vi "ALR ON_OFFs.vi"(8 "error in (no error)":errorcluster, 9 "Data":bool[](array[boolean]), 10 "Index":i32[](array[numeric]), 11 "ALR_ON_OFF":T1) -> (0 "error out":errorcluster, 3 "ALR_ON_OFF out":T1)   [LabVIEW 2019, in "Alarms.lvlib"]
uses:
  Alarms.lvlib
  Ctl/ALR_ON_OFF.ctl
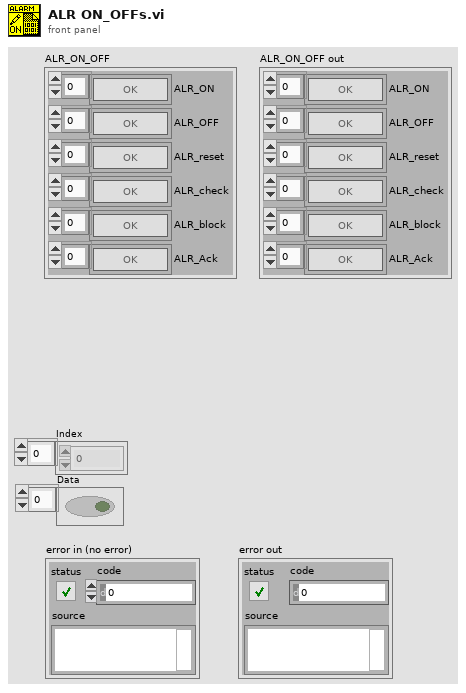
[diagram p1: front panel]
types:
  T1 = typedef "Alarms.lvlib/ALR_ON_OFF.ctl" = cluster{"ALR_ON":bool[], "ALR_OFF":bool[], "ALR_reset":bool[], "ALR_check":bool[], "ALR_block":bool[], "ALR_Ack":bool[]}
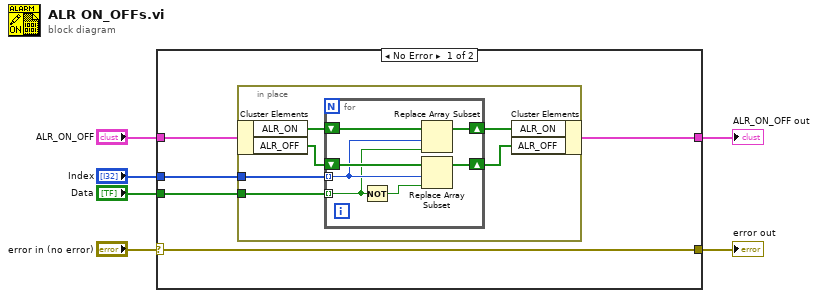
[diagram p0: block diagram]
diagram:
  n1 = case shown="No Error" "error in (no error)" {
    selector: "error in (no error)" -> [w8 w26]
    tunnel: "Index" -> [w11 _]
    tunnel: [w8 w26] -> w5
    tunnel: "ALR_ON_OFF" -> [w9 w25]
    tunnel: "Data" -> [w10 _]
    tunnel: [w7 w25] -> w1
    frame No Error {
      n2 = in-place {
        in-place-border: w11 -> [w16]
        in-place-border: w10 -> [w14]
        n3 = in-place-cluster #1(w9) -> ("ALR_ON"=w17:bool[], "ALR_OFF"=w15:bool[])
        n4 = for {
          tunnel: w16 -> [w22] mode=indexing
          tunnel: w14 -> [w21] mode=indexing
          shift-right: [w20] -> w13
          shift-left: w17 -> [w24]
          shift-right: [w19] -> w12
          shift-left: w15 -> [w23]
          n5 = Not(x=w21) -> (.not. x?=w18:bool)
          n6 = Replace Array Subset(array=w24, new element=w21, index=w22) -> (w20:bool[])
          n7 = Replace Array Subset(array=w23, new element=w18, index=w22) -> (w19:bool[])
        }
        n8 = in-place-cluster #1("ALR_ON"=w13, "ALR_OFF"=w12) -> (w7:T1)
      }
    }
    frame Error {
    }
  }
  "error out" <- w5
  "ALR_ON_OFF out" <- w1
